vi "Cross.vi"(11 "Min/Max Voltage":dbl format="%#_13g") -> (0 "Rate":dbl=68200.0, 2 "Scanners trajectories":dbl[][](graph)=[[0.0, 0.003925413946193441, 0.007841371226364848, 0.01173843795642894, 0.015607225761290262, 0.019438414392261114, 0.02322277418035699, 0.02695118827137761, 0.030614674589207184, 0.03420440747442258, 0.03771173894607982, 0.04112821953545775, 0.04444561864156819, 0.04765594435939468, 0.050751462733091654, 0.05372471638776148, 0.05656854249492382, 0.05927609002839673, 0.06184083626901897, 0.0642566025184516, 0.06651756898420363, 0.06861828880002177, 0.07055370114786842, 0.07231914344987547, 0.07391036260090296, 0.07532352521464167, 0.07655522685857673, 0.07760250025556352, 0.07846282243225845, 0.07913412079718248, 0.07961477813377577, 0.07990363649641379, 0.08, 0.07990363649641379, 0.07961477813377575, 0.07913412079718248, 0.07846282243225844, 0.07760250025556352, 0.07655522685857671, 0.07532352521464167, 0.07391036260090295, 0.07231914344987547, 0.07055370114786841, 0.06861828880002177, 0.06651756898420362, 0.0642566025184516, 0.061840836269018956, 0.05927609002839673, 0.0565685424949238, 0.05372471638776148, 0.05075146273309164, 0.04765594435939468, 0.04444561864156818, 0.04112821953545775, 0.03771173894607981, 0.03420440747442258, 0.030614674589207184, 0.026951188271377612, 0.023222774180356995, 0.01943841439226112, 0.01560722576129027, 0.011738437956428949, 0.007841371226364857, 0.003925413946193449, 1.0408340855860843e-17, -0.0039254139461934335, -0.007841371226364836, -0.011738437956428933, -0.015607225761290248, -0.019438414392261107, -0.023222774180356974, -0.026951188271377602, -0.030614674589207164, -0.03420440747442256, -0.03771173894607979, -0.041128219535457734, -0.04444561864156816, -0.047655944359394665, -0.05075146273309162, -0.05372471638776147, -0.05656854249492378, -0.05927609002839672, -0.061840836269018935, -0.06425660251845158, -0.06651756898420359, -0.06861828880002176, -0.07055370114786838, -0.07231914344987546, -0.07391036260090292, -0.07532352521464165, -0.07655522685857669, -0.0776025002555635, -0.07846282243225841, -0.07913412079718246, -0.07961477813377572, -0.07990363649641377, -0.07999999999999997, -0.07990363649641377, -0.07961477813377572, -0.07913412079718246, -0.07846282243225841, -0.0776025002555635, -0.07655522685857669, -0.07532352521464165, -0.07391036260090292, -0.07231914344987546, -0.07055370114786838, -0.06861828880002176, -0.06651756898420359, -0.06425660251845158, -0.061840836269018935, -0.05927609002839672, -0.05656854249492378, -0.05372471638776147, -0.050751462733091626, -0.047655944359394665, -0.044445618641568166, -0.04112821953545774, -0.037711738946079806, -0.03420440747442257, -0.030614674589207178, -0.02695118827137761, -0.023222774180356988, -0.019438414392261117, -0.015607225761290264, -0.011738437956428947, -0.007841371226364855, -0.003925413946193451], [0.08, 0.0799036364964138, 0.07961477813377575, 0.07913412079718249, 0.07846282243225844, 0.07760250025556353, 0.07655522685857671, 0.07532352521464168, 0.07391036260090295, 0.07231914344987549, 0.07055370114786841, 0.06861828880002178, 0.06651756898420362, 0.06425660251845161, 0.061840836269018956, 0.05927609002839675, 0.0565685424949238, 0.053724716387761495, 0.05075146273309164, 0.04765594435939469, 0.04444561864156818, 0.04112821953545776, 0.03771173894607981, 0.03420440747442259, 0.030614674589207184, 0.026951188271377626, 0.02322277418035699, 0.019438414392261134, 0.015607225761290262, 0.011738437956428963, 0.00784137122636485, 0.003925413946193463, 1.734723475976807e-18, -0.00392541394619342, -0.007841371226364847, -0.01173843795642892, -0.015607225761290259, -0.019438414392261093, -0.023222774180356988, -0.026951188271377588, -0.03061467458920718, -0.03420440747442255, -0.03771173894607981, -0.04112821953545772, -0.04444561864156818, -0.04765594435939465, -0.05075146273309164, -0.053724716387761454, -0.0565685424949238, -0.059276090028396705, -0.061840836269018956, -0.06425660251845157, -0.06651756898420362, -0.06861828880002174, -0.07055370114786841, -0.07231914344987544, -0.07391036260090295, -0.07532352521464164, -0.07655522685857671, -0.07760250025556349, -0.07846282243225844, -0.07913412079718245, -0.07961477813377575, -0.07990363649641376, -0.08, -0.07990363649641376, -0.07961477813377575, -0.07913412079718245, -0.07846282243225844, -0.07760250025556349, -0.07655522685857671, -0.07532352521464164, -0.07391036260090295, -0.07231914344987544, -0.07055370114786841, -0.06861828880002174, -0.06651756898420362, -0.06425660251845157, -0.061840836269018956, -0.059276090028396705, -0.0565685424949238, -0.053724716387761454, -0.05075146273309164, -0.04765594435939465, -0.04444561864156818, -0.04112821953545773, -0.03771173894607981, -0.034204407474422556, -0.030614674589207184, -0.026951188271377595, -0.023222774180356995, -0.019438414392261103, -0.01560722576129027, -0.011738437956428933, -0.007841371226364857, -0.003925413946193437, -1.0408340855860843e-17, 0.003925413946193442, 0.007841371226364836, 0.011738437956428939, 0.015607225761290248, 0.019438414392261107, 0.023222774180356974, 0.0269511882713776, 0.030614674589207164, 0.03420440747442256, 0.03771173894607979, 0.041128219535457734, 0.04444561864156816, 0.04765594435939466, 0.05075146273309162, 0.05372471638776146, 0.05656854249492378, 0.05927609002839671, 0.061840836269018935, 0.06425660251845157, 0.06651756898420359, 0.06861828880002174, 0.07055370114786838, 0.07231914344987544, 0.07391036260090292, 0.07532352521464164, 0.07655522685857669, 0.07760250025556349, 0.07846282243225841, 0.07913412079718245, 0.07961477813377572, 0.07990363649641376]], 3 "XY Graph":cluster{dbl[], "Ramp Pattern":dbl[]}(graph))   [LabVIEW 2021]
doc: "This VI enables to display the Cross optotype.\n\nInput:\n(1) Min/Max Voltage - the absolute value of the Voltage. Due to this parameter, the size of the optotype can be changed. Voltage about 10V is not allowed.\n\nOutputs: \n(1) XY Graph - the optotype data, to display the pattern.\n(2) Scanners trajectories - the XY data for the Scanners.\n(3) Rate - the rate parameter equal to 68200."
uses:
  <vilib>/Analysis/1siggen.llb/Ramp Pattern by Samples.vi
  <vilib>/Analysis/NI_AALBase.lvlib
panel:
  in  "Samples in line":i32=200
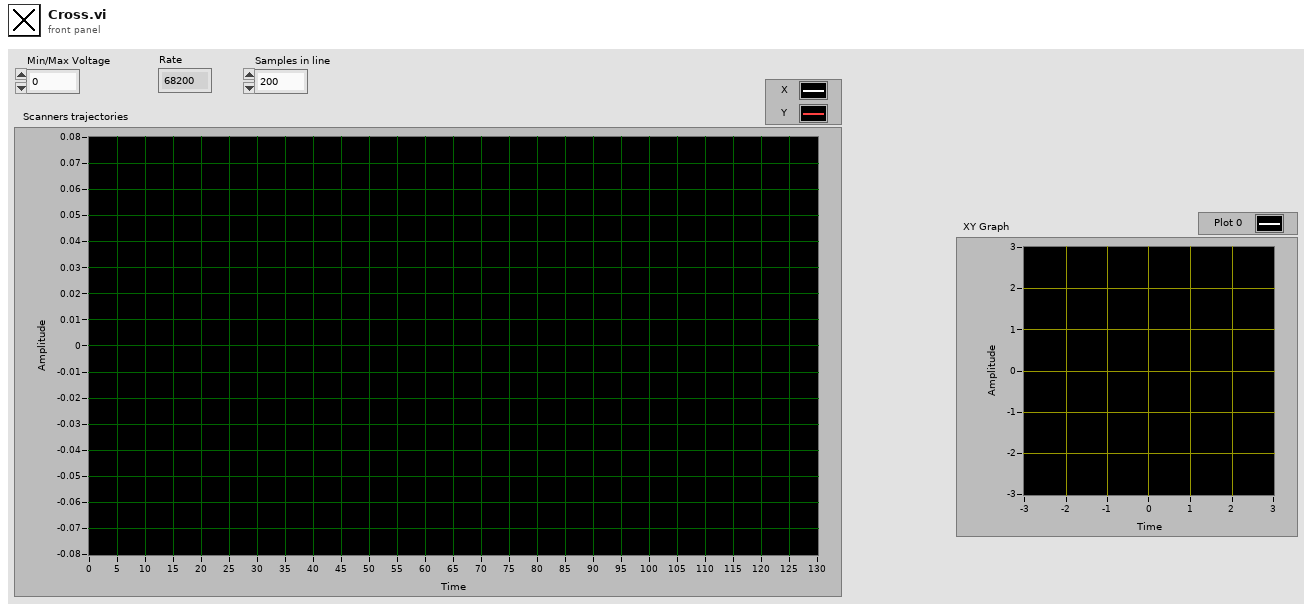
[diagram p1: front panel]
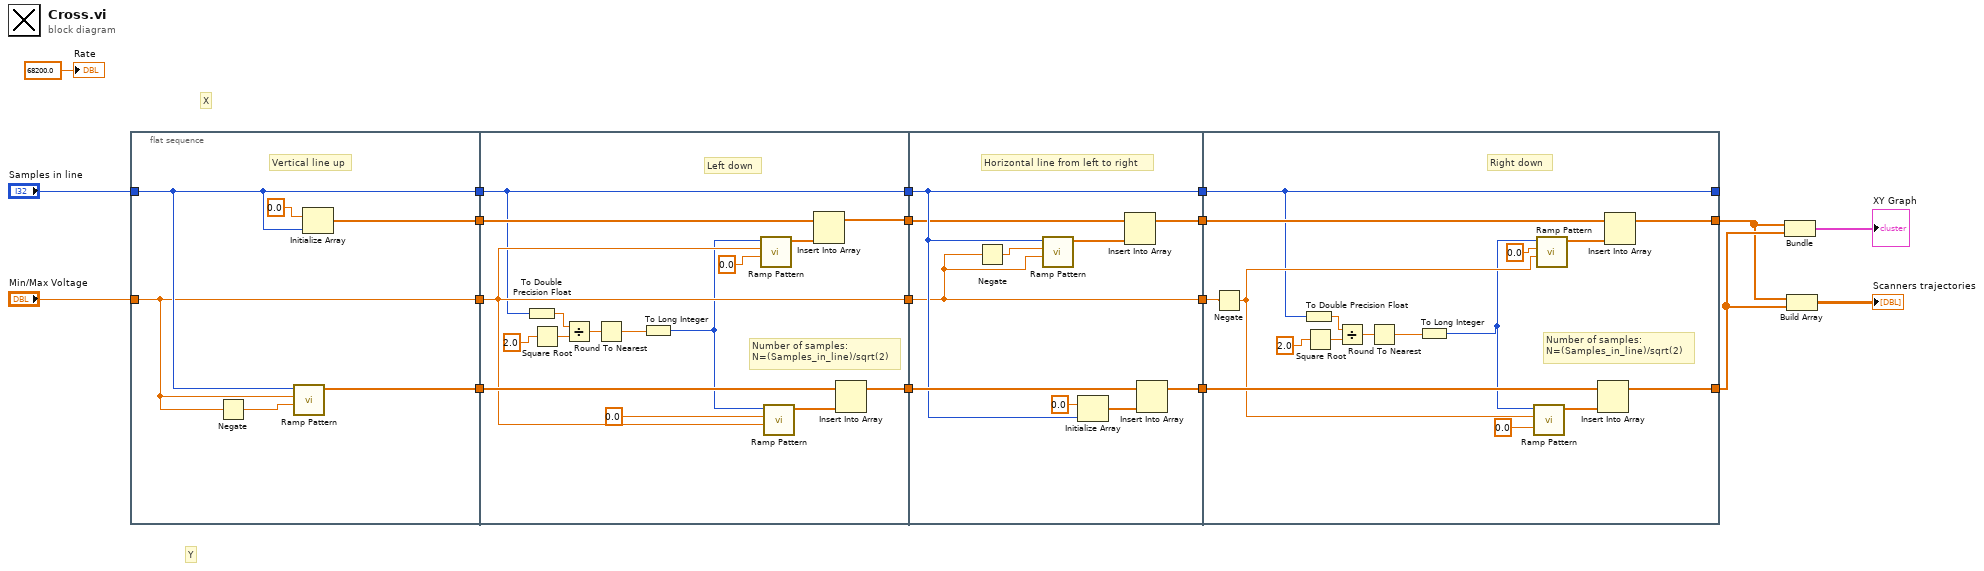
[diagram p0: block diagram]
diagram:
  # "Y"
  # "X"
  n1 = flat-sequence {
    tunnel: "Min/Max Voltage" -> [w22]
    tunnel: "Samples in line" -> [w23]
    tunnel: [w20] -> w16
    tunnel: [w23] -> w13
    tunnel: [w22] -> w10
    tunnel: [w21] -> w6
    tunnel: w16 -> [w40]
    tunnel: [w30] -> w15
    tunnel: w13 -> [w28]
    tunnel: [w39] -> w11
    tunnel: w10 -> [w39]
    tunnel: [w28] -> w8
    tunnel: [w36] -> w7
    tunnel: w6 -> [w34]
    tunnel: w15 -> [w49]
    tunnel: [w48] -> w14
    tunnel: [w42] -> w12
    tunnel: w11 -> [w42]
    tunnel: [w47] -> w9
    tunnel: w8 -> [w47]
    tunnel: w7 -> [w44]
    tunnel: [w45] -> w5
    tunnel: [w64] -> w3
    tunnel: w14 -> [w65]
    tunnel: w12 -> [w57]
    tunnel: [w52] -> _
    tunnel: w9 -> [w52]
    tunnel: [w62] -> w2
    tunnel: w5 -> [w61]
    frame #0 {
      # "Vertical line up"
      n2 = Negate(x=w22) -> (-x=w25:dbl)
      n3 = call-poly <vilib>:"Ramp Pattern.vi"("start"=w25, "end"=w22, "samples"=w23) -> ("Ramp Pattern"=w20:dbl[])  [unwired: 7 in, 1 out]
      n4 = Initialize Array(0.0 ("element"), w23) -> (w21:dbl[])
    }
    frame #1 {
      # "Left down"
      # "Number of samples:\nN=(Samples_in_line)/sqrt(2)"
      n5 = To Double Precision Float(number=w28) -> (double precision float=w29:dbl)
      n6 = Square Root(x=2.0) -> (sqrt(x)=w33:dbl)
      n7 = Divide(x=w29, y=w33) -> (x/y=w31:dbl)
      n8 = Round To Nearest(number=w31) -> (nearest integer value=w27:dbl)
      n9 = To Long Integer(number=w27) -> (32bit integer=w26:i32)
      n10 = call-poly <vilib>:"Ramp Pattern.vi"("start"=0.0, "end"=w39, "samples"=w26) -> ("Ramp Pattern"=w35:dbl[])  [unwired: 7 in, 1 out]
      n11 = call-poly <vilib>:"Ramp Pattern.vi"("start"=w39, "end"=0.0, "samples"=w26) -> ("Ramp Pattern"=w41:dbl[])  [unwired: 7 in, 1 out]
      n12 = Insert Into Array(array=w34, new element=w35) -> (w36:dbl[])  [unwired: 1 in]
      n13 = Insert Into Array(array=w40, new element=w41) -> (w30:dbl[])  [unwired: 1 in]
    }
    frame #2 {
      # "Horizontal line from left to right"
      n14 = Negate(x=w42) -> (-x=w43:dbl)
      n15 = call-poly <vilib>:"Ramp Pattern.vi"("start"=w42, "end"=w43, "samples"=w47) -> ("Ramp Pattern"=w46:dbl[])  [unwired: 7 in, 1 out]
      n16 = Initialize Array(0.0 ("element"), w47) -> (w50:dbl[])
      n17 = Insert Into Array(array=w44, new element=w46) -> (w45:dbl[])  [unwired: 1 in]
      n18 = Insert Into Array(array=w49, new element=w50) -> (w48:dbl[])  [unwired: 1 in]
    }
    frame #3 {
      # "Right down"
      # "Number of samples:\nN=(Samples_in_line)/sqrt(2)"
      n19 = Negate(x=w57) -> (-x=w56:dbl)
      n20 = To Double Precision Float(number=w52) -> (double precision float=w53:dbl)
      n21 = Square Root(x=2.0) -> (sqrt(x)=w68:dbl)
      n22 = Divide(x=w53, y=w68) -> (x/y=w66:dbl)
      n23 = Round To Nearest(number=w66) -> (nearest integer value=w55:dbl)
      n24 = To Long Integer(number=w55) -> (32bit integer=w54:i32)
      n25 = call-poly <vilib>:"Ramp Pattern.vi"("start"=0.0, "end"=w56, "samples"=w54) -> ("Ramp Pattern"=w63:dbl[])  [unwired: 7 in, 1 out]
      n26 = call-poly <vilib>:"Ramp Pattern.vi"("start"=w56, "end"=0.0, "samples"=w54) -> ("Ramp Pattern"=w60:dbl[])  [unwired: 7 in, 1 out]
      n27 = Insert Into Array(array=w65, new element=w63) -> (w64:dbl[])  [unwired: 1 in]
      n28 = Insert Into Array(array=w61, new element=w60) -> (w62:dbl[])  [unwired: 1 in]
    }
  }
  n29 = Bundle(w2, "Ramp Pattern"=w3) -> (→"XY Graph":cluster{dbl[], "Ramp Pattern":dbl[]})  [unwired: 1 in]
  n30 = Build Array(w2, w3) -> (→"Scanners trajectories":dbl[][])
  "Rate" <- 68200.0
